vi "LoadZlut.vi"() -> ()   [LabVIEW 2011]
panel:
  out "Intensity Graph":dbl[][](graph)
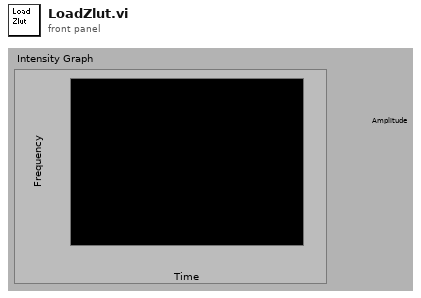
[diagram p1: front panel]
types:
  T1 = enum16{"init", "get", "set single frame", "set all"}
  T2 = cluster{"ROI1":i32, "Rmax (pix)":i32, "RminZ (pix)":i32, "LUTs":dbl[][][], "use trace":bool, "angular pixel\n coverage factor":dbl, "radial pixel\n coverage factor":dbl}
  T3 = typedef "IMAQ Image.ctl" = refnum<image>
  T4 = cluster{"front panel settings":cluster{"files":cluster{"LUT path":path, "Trace path":path, " folders #":i32, "base path":path, "use trace":bool, "use base":bool, "LUT tmp":i32, "Trace tmp":i32, "active path":path}, "Tracking":cluster{"RminZ (pix)":i32, "Rmax (pix)":i32, "angular pixel \ncoverage factor":dbl, "radial pixel \ncoverage factor":dbl}, "Frames":cluster{"Start frame":i32, "number of frames":u32, "display frame ":i32, "track every nd frame ":i32, "Track all frames":bool, "active frame":i32}, "Calibs":cluster{"Zlut number of steps":i32, "pix/um":dbl, "Z correction factor":dbl, "Zlut step size (um)":dbl, "ROI(pix)":i32}, "Beads":cluster{"number of ref beads":i32, "overlay":bool}, "Misc":cluster{"save images to new location":bool, "destination":path}}, "data":cluster{"Image":T3, "image size":i32[], "Bead Array":i32[][], "overlay image":T3, "# beads":i32, "Job list":string[][], "job running":bool, "job #":i32, "folders to go":i32}}
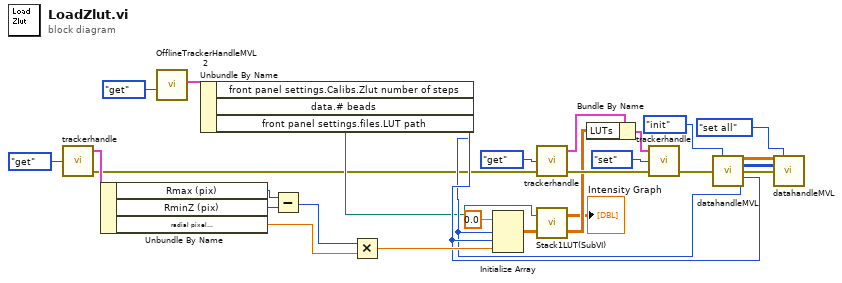
[diagram p0: block diagram]
diagram:
  n1 = call "trackerhandle.vi"("action"=enum16{"get", "set"}."get") -> ("error out"=w1:errorcluster, "output Cluster"=w17:T2)  [unwired: 2 in, 1 out]
  n2 = Unbundle By Name(w17) -> ("Rmax (pix)"=w12:i32, "RminZ (pix)"=w11:i32, "radial pixel\n coverage factor"=w7:dbl)
  n3 = call "OfflineTrackerHandleMVL2.vi"("action"=enum16{"get", "set"}."get") -> ("out"=w5:T4)  [unwired: 5 in, 1 out]
  n4 = Unbundle By Name(w5) -> ("front panel settings.Calibs.Zlut number of steps"=w4:i32, "data.# beads"=w3:i32, "front panel settings.files.LUT path"=w2:path)
  n5 = Subtract(x=w12, y=w11) -> (x-y=w10:i32)
  n6 = Multiply(x=w10, y=w7) -> (x*y=w9:dbl)
  n7 = Initialize Array(0.0 ("element"), w3, w4, w9) -> (w19:dbl[][][])
  n8 = call "trackerhandle.vi"("error in"=w1, "action"=enum16{"get", "set"}."get") -> ("error out"=w16:errorcluster, "output Cluster"=w22:T2)  [unwired: 1 in, 1 out]
  n9 = call "Stack1LUT(SubVI).vi"("Array"=w19, "LUT image data path 2"=w2) -> ("Stacked LUTs"=w14:dbl[][][], "Intensity Graph"=→"Intensity Graph":dbl[][])
  n10 = Bundle By Name(cluster=w22, "LUTs"=w14) -> (w21:T2)
  n11 = call "trackerhandle.vi"("error in"=w16, "action"=enum16{"get", "set"}."set", "input Cluster"=w21) -> ("error out"=w15:errorcluster)  [unwired: 2 out]
  n12 = call "datahandleMVL.vi"("action"=T1."init", "error in"=w15, "number of frames"=w4, "number of beads"=w3) -> ("XYZ out"=w28:dbl[][][], "time out"=w27:i32[][], "error in 2"=w26:errorcluster)  [unwired: 6 in, 3 out]
  n13 = call "datahandleMVL.vi"("xyz array in"=w28, "action"=T1."set all", "Time array in"=w27, "error in"=w26) -> ()  [unwired: 6 in, 6 out]
